vi "Pre Launch Init.vi"(11 "Stage in":refnum<class "Stage.lvclass">) -> (0 "error out":errorcluster, 3 "Stage out":refnum<class "Stage.lvclass">)   [LabVIEW 2020, in "Stage.lvlib" / "Stage.lvclass"]
doc: "(<B>Filename</B>: Actor Framework.lvlib:Actor.lvclass:Pre Launch Init.vi)\n\nDefines behavior that occurs after the Launch Nested Actor method is invoked but before the actor's Actor Core method begins running.\n\nBy default, this method does nothing. A descendant class may override it to define behavior."
uses:
  Stage.lvclass
  Device/Device/Device.lvclass
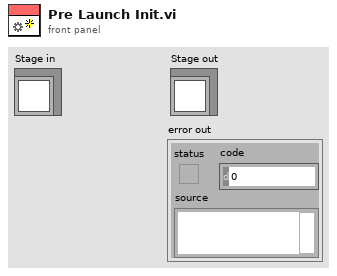
[diagram p1: front panel]
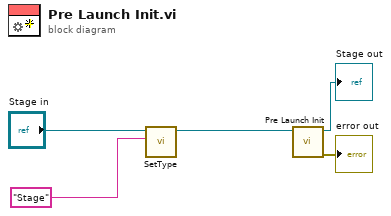
[diagram p0: block diagram]
diagram:
  n1 = call-dynamic "SetType.vi"("Type"="Stage", "Device in"="Stage in") -> ("Device out"=w2:refnum<class "Stage.lvclass">)  [unwired: 8 in, 1 out]
  n2 = call-parent "Pre Launch Init.vi"("Device in"=w2) -> ("error out"=→"error out":errorcluster, "Device out"=→"Stage out":refnum<class "Stage.lvclass">)  [unwired: 9 in]
